vi "Configure Standard Waveform Advanced (Ramp).vi"(8 "error in (no error)":errorcluster, 9 "Ramp Symmetry (100 Percent)":dbl=100.0, 10 "Channel (1: 1)":u16(ring)=1 items=["1"=1, "2"=2], 11 "VISA resource name":refnum<visa-resource-name>) -> (0 "error out":errorcluster, 3 "VISA resource name out":refnum<visa-resource-name>)   [LabVIEW 2023, in "Keysight-33500B.lvlib"]
doc: "Sets symmetry percent for ramp waveform.\nSymmetry represents the amount of time per cycle that the ramp wave is rising (assuming that the waveform polarity is not inverted).\n\n<b>Note</b>:\n(1) This VI is only used to work with Configure Standard Waveform.VI when waveform function is set to RAMP\n(2) The symmetry setting is remembered when you change from ramp wave to another function. When you return to the ramp wave function, the previous symmetry is used. \n(3) If you select a ramp waveform as the modulating waveform for AM or FM, the symmetry setting does not apply. The waveform generator always uses a ramp waveform with a 100% duty cycle."
uses:
  Keysight-33500B.lvlib
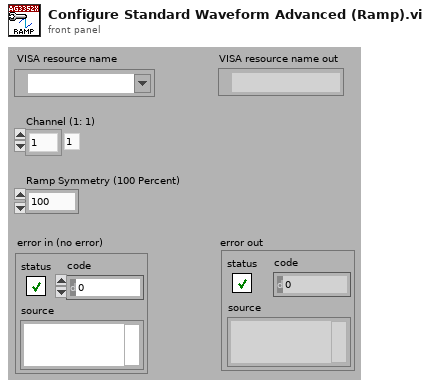
[diagram p1: front panel]
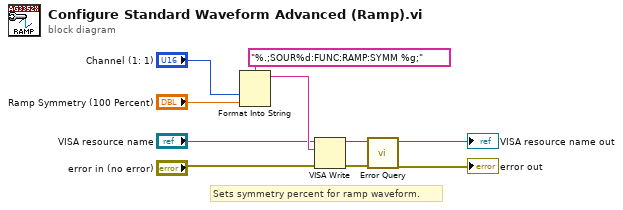
[diagram p0: block diagram]
diagram:
  # "Sets symmetry percent for ramp waveform."
  n1 = Format Into String(format string="%.;SOUR%d:FUNC:RAMP:SYMM %g;", "Channel (1: 1)", "Ramp Symmetry (100 Percent)") -> (resulting string=w7:string)  [unwired: 2 in, 1 out]
  n2 = VISA Write(VISA resource name="VISA resource name", write buffer=w7, error in (no error)="error in (no error)") -> (VISA resource name out=w4:refnum<visa-resource-name>, error out=w3:errorcluster)  [unwired: 1 out]
  n3 = call "Error Query.vi"("error in (no error)"=w3, "VISA resource name"=w4) -> ("error out"=→"error out":errorcluster, "VISA resource name out"=→"VISA resource name out":refnum<visa-resource-name>)  [unwired: 8 out]
